vi "catch file exception.vi"(8 "exception in":T3 {"code" format="%.0x"}) -> (0 "exception out":T3 {"code" format="%.0x"}, 1 "severity":T2, 2 "file error":T1, 3 "file exception?":bool, 5 "file exception":T3 {"code" format="%.0x"})   [LabVIEW 2013, in "file errors.lvlib"]
uses:
  file errors.lvlib
  exception.ctl
  severity.ctl
  file error.ctl
  exception.lvlib
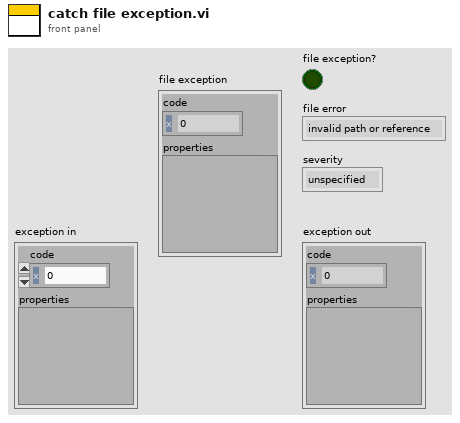
[diagram p1: front panel]
types:
  T1 = typedef "file errors.lvlib/file error.ctl" = enum16{"invalid path or reference", "end of file", "file already opened", "generic file error", "file not found", "permissions invalid", "disk full", "duplicate path", "too many open file handles", "useless generic error"}
  T2 = typedef "exception.lvlib/severity.ctl" = enum8{"unspecified", "informational", "operation failed", "data corruption", "system corruption", "critical unknown state"}
  T3 = typedef "exception.lvlib/exception.ctl" = cluster{"code":i32, "properties":variant}
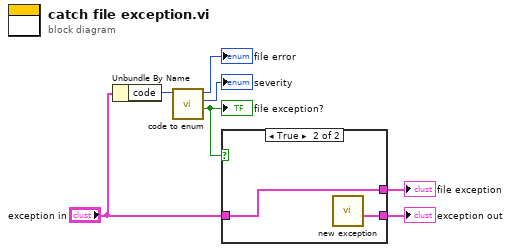
[diagram p0: block diagram]
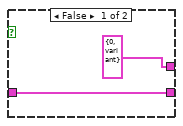
[diagram p2: hidden frame]
diagram:
  n1 = Unbundle By Name("exception in") -> ("code"=w7:i32)
  n2 = call "code to enum.vi"("code"=w7) -> ("valid?"=w6:bool, "severity"=→"severity":T2, "file error"=→"file error":T1)  [unwired: 8 in]
  "file exception?" <- w6
  n3 = case shown="True" w6 {
    tunnel: "exception in" -> [w9 w11]
    tunnel: [T3 {"code"=0, "properties"=variant} ("exception in") w11] -> w4
    tunnel: [w9 w10] -> w1
    frame False {
    }
    frame True {
      n4 = call "new exception.vi"() -> ("exception"=w10:T3)  [unwired: 11 in]
    }
  }
  "exception out" <- w1
  "file exception" <- w4
